vi "12.Evd.5_Ask.1.vi"() -> ()   [LabVIEW 2025]
panel:
  in  "stop":bool
  out "Result":dbl
  in  "Boolean":bool=TRUE
  in  "B":dbl
  in  "A":dbl
  # "Add"
  # "Sub"
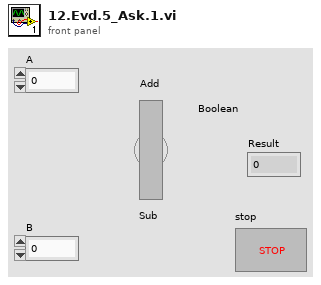
[diagram p1: front panel]
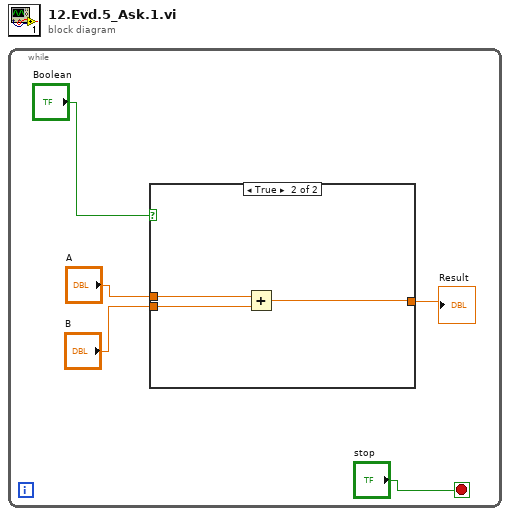
[diagram p0: block diagram]
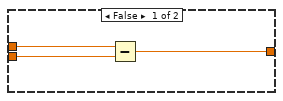
[diagram p2: hidden frame]
diagram:
  n1 = while {
    stop <- "stop" stop-if-true
    n2 = case shown="True" "Boolean" {
      tunnel: "A" -> [w8 w11]
      tunnel: "B" -> [w7 w10]
      tunnel: [w6 w9] -> w1
      frame False {
        n3 = Subtract(x=w8, y=w7) -> (x-y=w6:dbl)
      }
      frame True {
        n4 = Add(x=w11, y=w10) -> (x+y=w9:dbl)
      }
    }
    "Result" <- w1
  }
